vi "Scripting.vi"() -> ()   [LabVIEW 2015]
uses:
  Utils/Cluster.ctl
  <vilib>/Utility/file.llb/Read Delimited Spreadsheet (string).vi
  Users/Sherman/Desktop/BETA_GSCS/Systems/TCS_Link/TCSLINK_global.vi
panel:
  out "Current Lamp cluster":T1
  out "Current Setup Name":string
  out "Setup Names":string[](array[string])
  out "Length of script":dbl
  in  "Script":T2
  out "TCP Response":string
  in  "TCP Connection ID":refnum<k5>
  in  "Current Slit":string
  out "Current Target":cluster{"RA":string, "DEC":string}={"RA"="-00:00:00.00", "DEC"="-00:00:00.00"}
  in  "Custom ROI":cluster{i32, i32, i32, i32, i32, i32}[](array[cluster])
  out "Total Cluster":T3(array[cluster]) {"Configuration"."Select Mode:" items=["Custom", "Imaging", "300 All", "600 UV", "600 Blue", "600 Mid", "600 Red", "1200 m0", "1200 m1", "1200 m2", "1200 m3", "1200 m4", "1200 m5", "1200 m6", "1200 m7", "1200 RESOLVE", "400 m1", "400 m2", "930 m1", "930 m2", "930 m3", "930 m4", "930 m5", "930 m6", "400WD", "930TP", "400Fermi", "400Padgett", "400Lewis", "400Crotts", "600BLee", "600RLee", "400WW"]; "SI camera info"."DomePercent" min=0 step=1; "SI camera info"."Quartz Percent" min=0 step=1; "SI camera info"."CCD Readout Speed" items=["750 kHz, ATTN 0", "750 kHz, ATTN 2", "344 kHz, ATTN 0", "344 kHz, ATTN 3", "100 kHz, ATTN 2", "100 kHz, ATTN 3"]; "SI camera info"."CCD ROI Mode" items=["Imaging, 1x1  "=0, "Imaging, 2x2"=1, "Imaging, 3x3"=2, "Spectroscopic, 1x1"=3, "Spectroscopic, 2x2"=4, "Spectroscopic, 3x3"=5, "MOS, 1x1"=11, "MOS, 2x2"=12, "MOS, 3x3"=13, "Slicer"=6, "Spectroscopic, ZZ Ceti"=14, "Slit Imaging/Alignment"=7, "MOS Imaging/Alignment"=10, "Set user-defined ROI..."=21, "Custom Mode"=9]; "SI camera info"."Number of Exp" min=0 step=1; "SI camera info"."Exp time" min=0 step=1}
  in  "?":T4(tab)
  in  "Shutdown":bool
  in  "Test":bool
  in  "ABORT":bool
  in  "Pause Button":bool
  out "Current Line":dbl caption="Current LIne"
  in  "Make Script":bool
  out "status":string
  in  "Script location":path
  in  "Scripting Active":bool
  out "Runtime":dbl caption="Expected Runtime"
  out "Array":string[](array[string])
  out "Wavelength Mode":string
  out "Secondary Filter":string
  out "Primary Filter":string
  out "Slit":string
  out "Grating":string
  out "Camera Focus":dbl
  out "Grating Angle":dbl
  out "Camera Angle":dbl
  out "Coll Position":dbl
  in  "Get System Info":bool
  in  "Setups":T5(array[cluster])
  # "Eventually Add tcp response to a new tab"
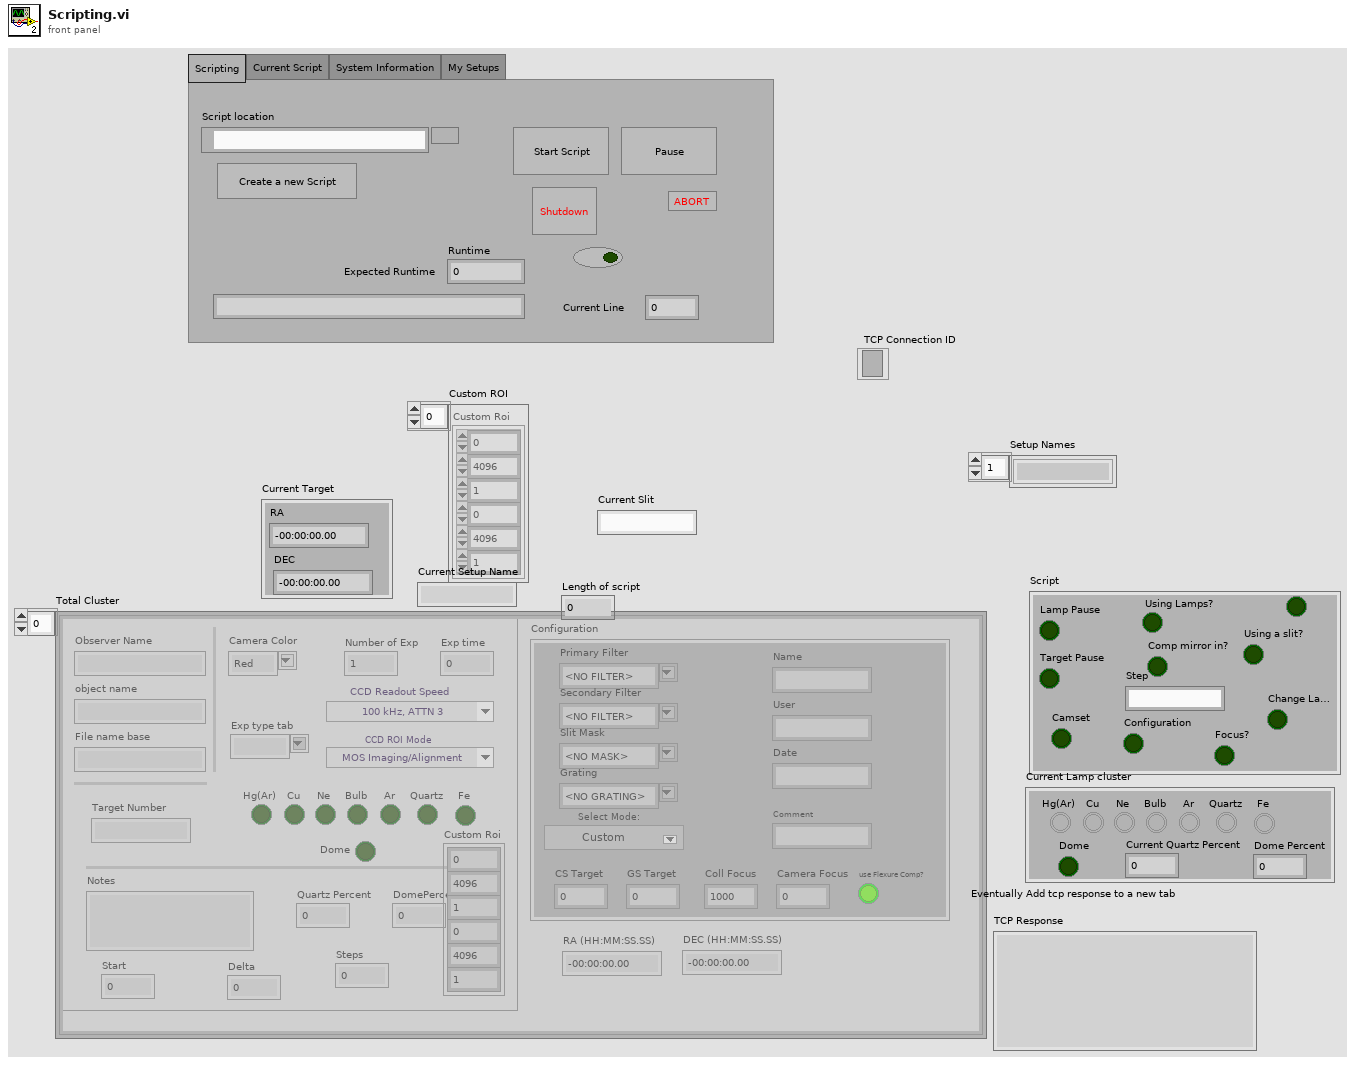
[diagram p1: front panel]
types:
  T1 = cluster{"Bulb":bool, "Fe":bool, "Quartz":bool, "Ar":bool, "Ne":bool, "Cu":bool, "Hg(Ar)":bool, "Current Quartz Percent":dbl, "Dome":bool, "Dome Percent":dbl}
  T2 = cluster{"Lamp Pause":bool, "Target Pause":bool, "Using Lamps?":bool, "Step":string, "Camset":bool, "Configuration":bool, "Using a slit?":bool, "Change Lamps":bool, "Boolean":bool, "Comp mirror in?":bool, "Focus?":bool}
  T3 = cluster{"SI camera info":cluster{"Observer Name":string, "object name":string, "File name base":string, "Camera Color":string, "Exp type tab":string, "Number of Exp":i32, "Exp time":i32, "CCD Readout Speed":u8, "CCD ROI Mode":u16, "Hg(Ar)":bool, "Cu":bool, "Ne":bool, "Bulb":bool, "Ar":bool, "Quartz":bool, "Quartz Percent":i32, "Fe":bool, "Notes":string, "Target Number":string, "DomePercent":i32, "Dome":bool, "Start":dbl, "Delta":dbl, "Steps":dbl, "Custom Roi":cluster{i32, i32, i32, i32, i32, i32}}, "Configuration":cluster{"Primary Filter":string, "Secondary Filter":string, "Slit Mask":string, "Grating":string, "CS Target":dbl, "GS Target":dbl, "Coll Focus":i32, "Camera Focus":i32, "Name":string, "User":string, "Date":string, "Comment":string, "use Flexure Comp?":bool, "Select Mode:":u16}, "RA (HH:MM:SS.SS)":string, "DEC (HH:MM:SS.SS)":string}[]
  T4 = enum32{"Scripting", "Current Script", "System Information", "My Setups"}
  T5 = cluster{"Setup Name":string, "Focus Value":dbl, "Focus Test updated?":bool}[]
  T6 = typedef "Cluster.ctl" = cluster{"SI camera info":cluster{"Observer Name":string, "object name":string, "File name base":string, "Camera Color":string, "Exp type tab":string, "Number of Exp":i32, "Exp time":i32, "CCD Readout Speed":u8, "CCD ROI Mode":u16, "Hg(Ar)":bool, "Cu":bool, "Ne":bool, "Bulb":bool, "Ar":bool, "Quartz":bool, "Quartz Percent":i32, "Fe":bool, "Notes":string, "Target Number":string, "DomePercent":i32, "Dome":bool, "Start":dbl, "Delta":dbl, "Steps":dbl, "Custom Roi":cluster{i32, i32, i32, i32, i32, i32}}, "Configuration":cluster{"Primary Filter":string, "Secondary Filter":string, "Slit Mask":string, "Grating":string, "CS Target":dbl, "GS Target":dbl, "Coll Focus":i32, "Camera Focus":i32, "Name":string, "User":string, "Date":string, "Comment":string, "use Flexure Comp?":bool, "Select Mode:":u16}, "RA (HH:MM:SS.SS)":string, "DEC (HH:MM:SS.SS)":string}
  T7 = cluster{"Setup Name":string, "Camera Focus":dbl, "Focus test updated?":bool}
  T8 = cluster{"SI camera info":cluster{"Observer Name":string, "object name":string, "File name base":string, "Camera Color":string, "Exp type tab":string, "Number of Exp":i32, "Exp time":i32, "CCD Readout Speed":u8, "CCD ROI Mode":u16, "Hg(Ar)":bool, "Cu":bool, "Ne":bool, "Bulb":bool, "Ar":bool, "Quartz":bool, "Quartz Percent":i32, "Fe":bool, "Notes":string, "Target Number":string, "DomePercent":i32, "Dome":bool, "Start":dbl, "Delta":dbl, "Steps":dbl, "Custom Roi":cluster{i32, i32, i32, i32, i32, i32}}, "Configuration":cluster{"Primary Filter":string, "Secondary Filter":string, "Slit Mask":string, "Grating":string, "CS Target":dbl, "GS Target":dbl, "Coll Focus":i32, "Camera Focus":i32, "Name":string, "User":string, "Date":string, "Comment":string, "use Flexure Comp?":bool, "Select Mode:":u16}, "RA (HH:MM:SS.SS)":string, "DEC (HH:MM:SS.SS)":string}
  T9 = cluster{"Setup Name":string, "Focus Value":dbl, "Focus Test updated?":bool}
  T10 = cluster{"Primary Filter":string, "Secondary Filter":string, "Slit Mask":string, "Grating":string, "CS Target":dbl, "GS Target":dbl, "Coll Focus":i32, "Camera Focus":i32, "Name":string, "User":string, "Date":string, "Comment":string, "use Flexure Comp?":bool, "Select Mode:":u16}
  T11 = cluster{"Observer Name":string, "object name":string, "File name base":string, "Camera Color":string, "Exp type tab":string, "Number of Exp":i32, "Exp time":i32, "CCD Readout Speed":u8, "CCD ROI Mode":u16, "Hg(Ar)":bool, "Cu":bool, "Ne":bool, "Bulb":bool, "Ar":bool, "Quartz":bool, "Quartz Percent":i32, "Fe":bool, "Notes":string, "Target Number":string, "DomePercent":i32, "Dome":bool, "Start":dbl, "Delta":dbl, "Steps":dbl, "Custom Roi":cluster{i32, i32, i32, i32, i32, i32}}
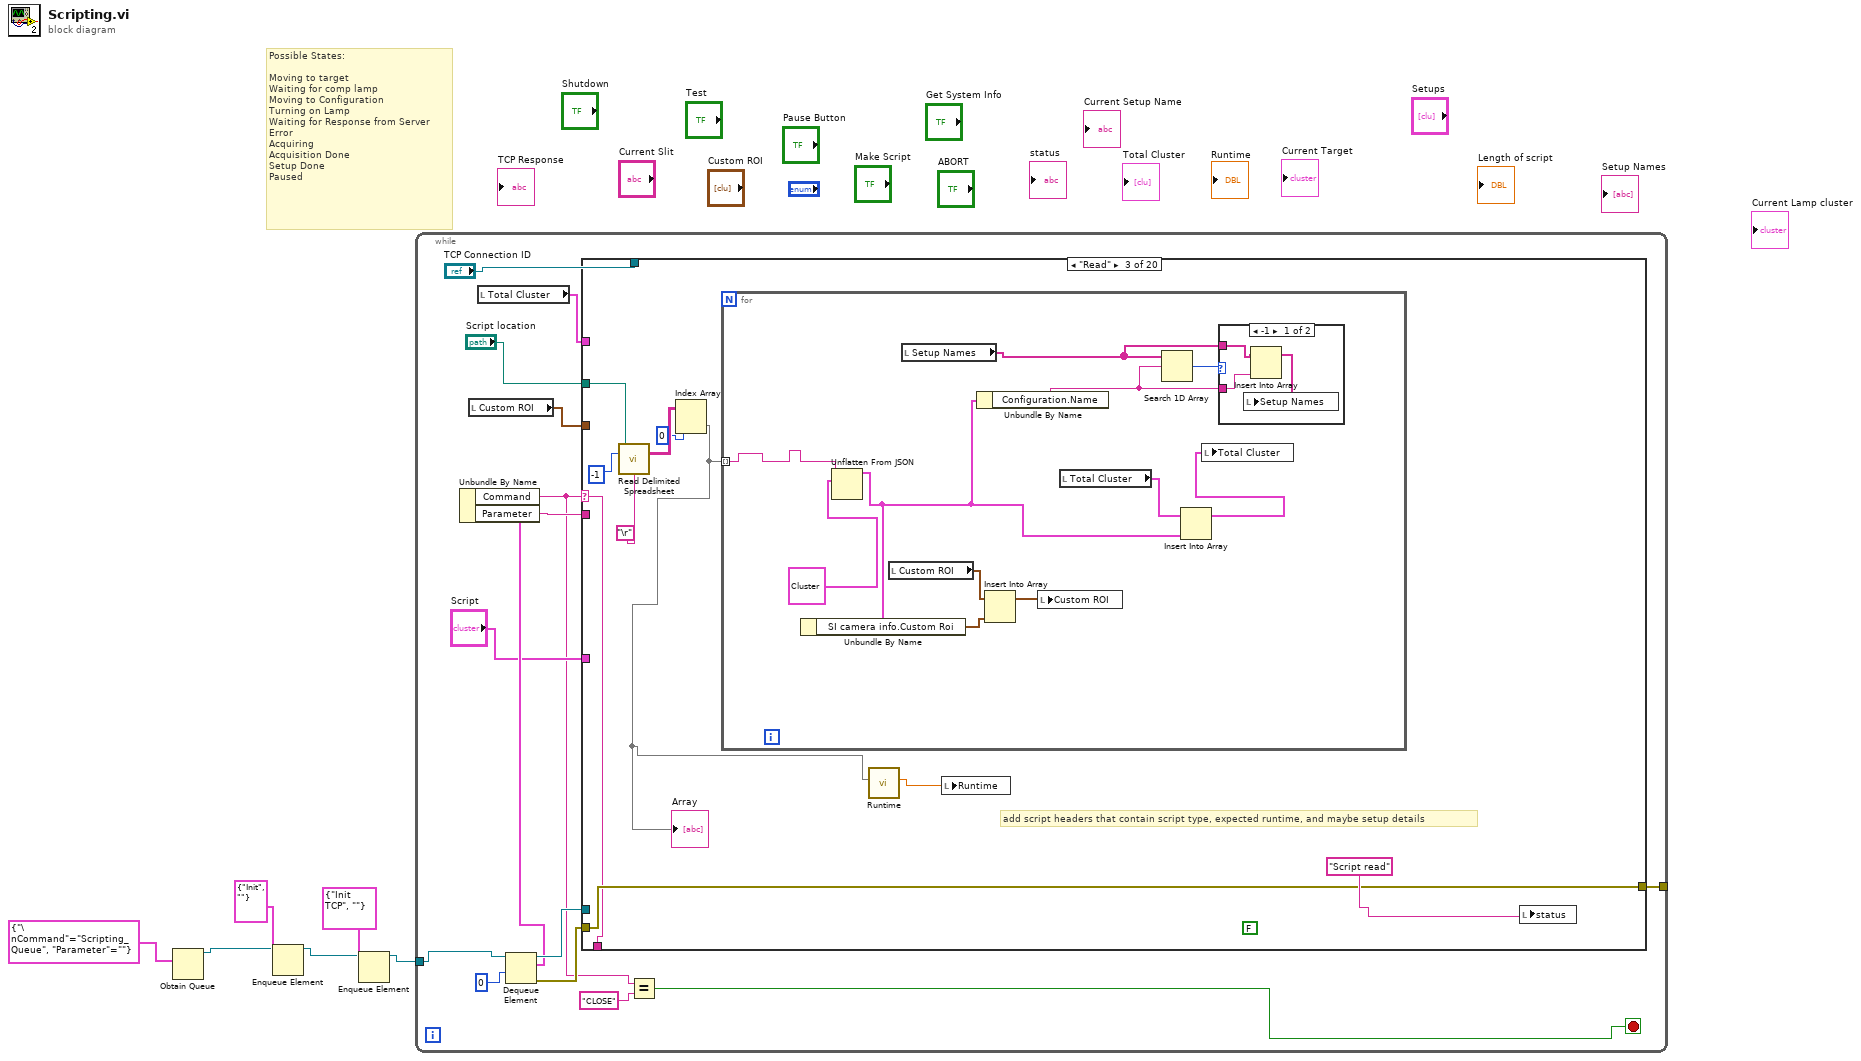
[diagram p0: block diagram]
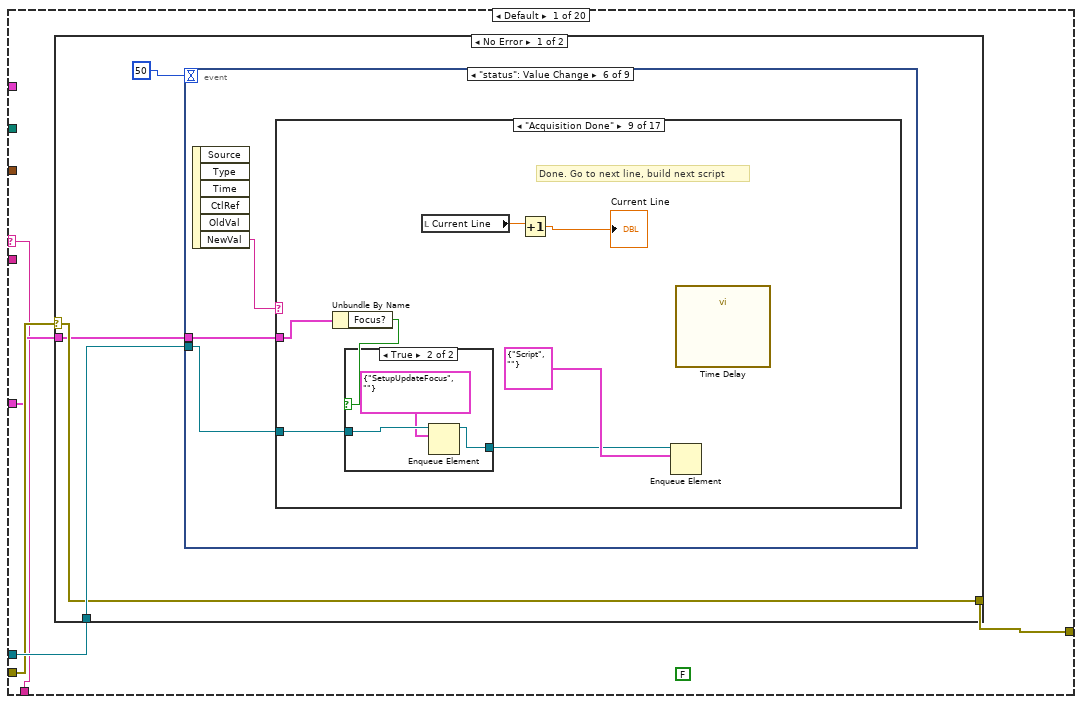
[diagram p2: hidden frame]
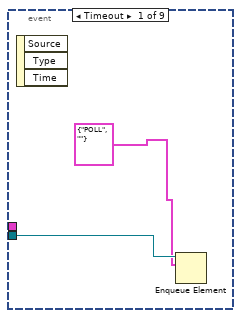
[diagram p3: hidden frame]
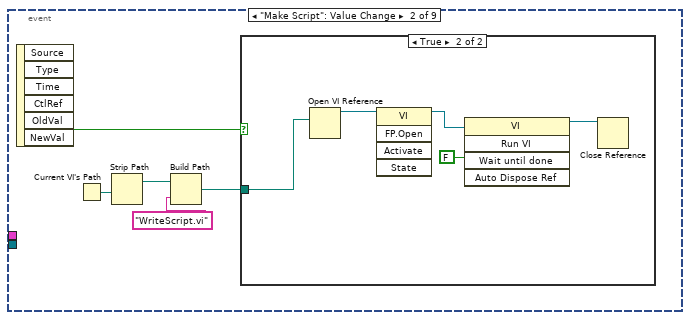
[diagram p4: hidden frame]
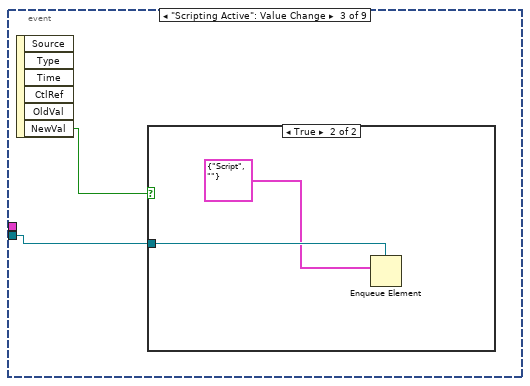
[diagram p6: hidden frame]
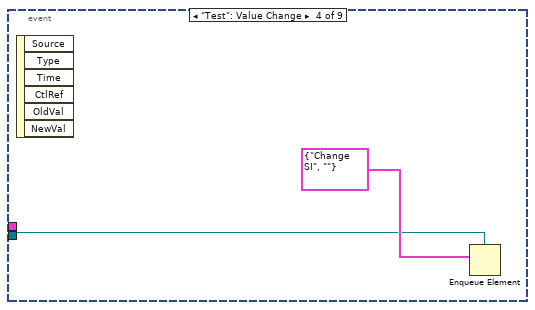
[diagram p8: hidden frame]
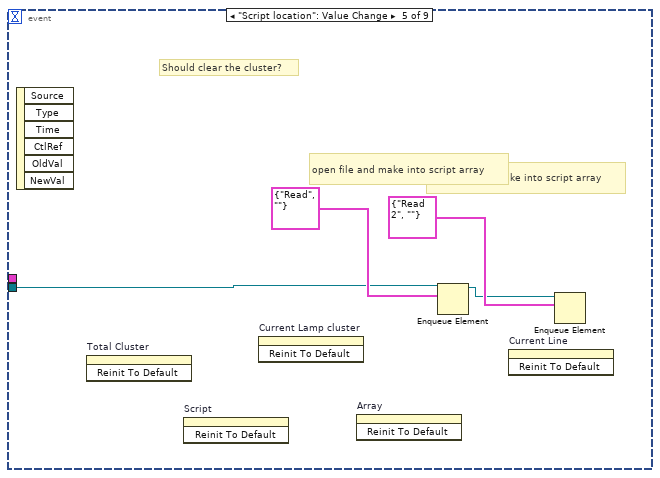
[diagram p9: hidden frame]
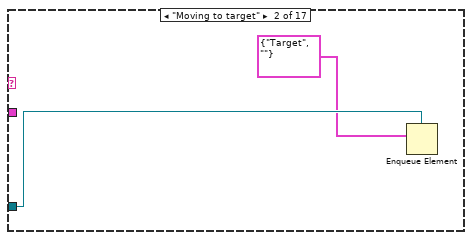
[diagram p11: hidden frame]
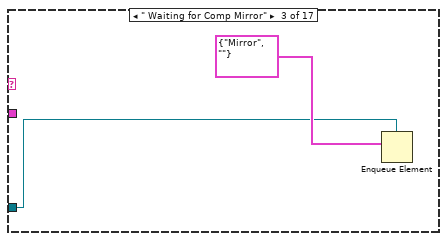
[diagram p12: hidden frame]
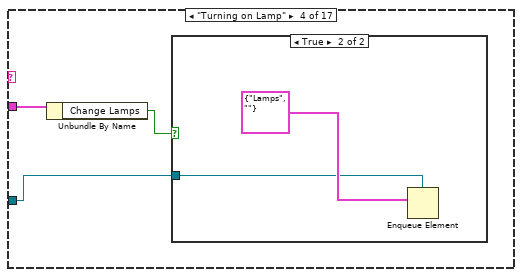
[diagram p13: hidden frame]
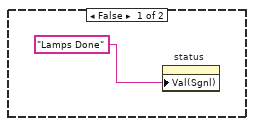
[diagram p14: hidden frame]
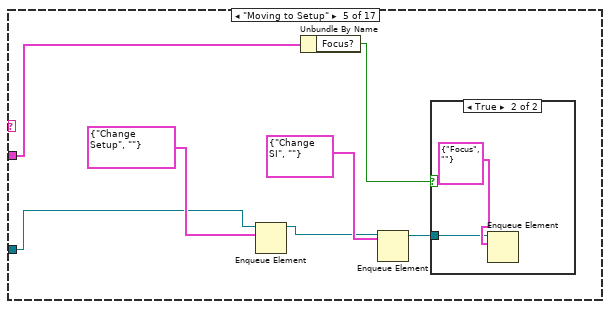
[diagram p15: hidden frame]
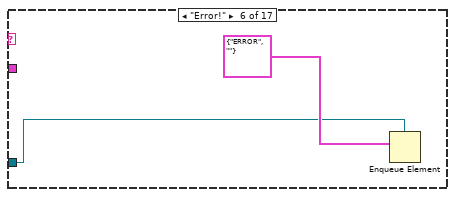
[diagram p17: hidden frame]
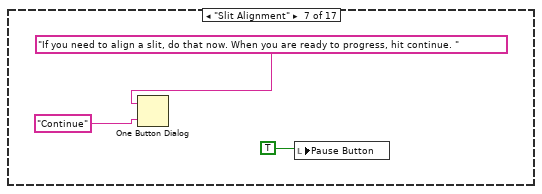
[diagram p18: hidden frame]
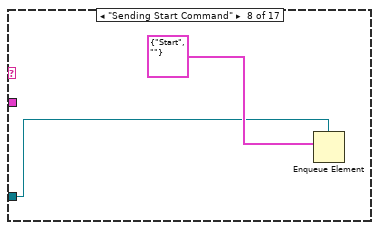
[diagram p19: hidden frame]
diagram:
  # "Possible States:\n\nMoving to target\nWaiting for comp lamp\nMoving to Configuration\nTurning on Lamp\nWaiting for Response from Server\nError\nAcquiring\nAcquisition Done\nSetup Done\nPaused"
  n1 = Obtain Queue(element data type=cluster{"\nCommand":string, "Parameter":string} {"\nCommand"="Scripting_Queue", "Parameter"=""}) -> (queue out=w2:refnum<queue>)  [unwired: 4 in, 2 out]
  n2 = Enqueue Element(queue=w2, element=cluster{string, string} {"Init", ""}) -> (queue out=w1:refnum<queue>)  [unwired: 2 in, 2 out]
  n3 = Enqueue Element(queue=w1, element=cluster{string, string} {"Init TCP", ""}) -> (queue out=w4:refnum<queue>)  [unwired: 2 in, 2 out]
  n4 = while {
    tunnel: w4 -> [w16]
    tunnel: [w11] -> _
    stop <- w7 stop-if-true
    n5 = local read "Custom ROI"() -> (w14:cluster{i32, i32, i32, i32, i32, i32}[])
    n6 = local read "Total Cluster"() -> (w17:T3)
    n7 = Dequeue Element(queue=w16, timeout in ms (-1)=0) -> (queue out=w21:refnum<queue>, element=w20:cluster{"\nCommand":string, "Parameter":string}, error out=w12:errorcluster)  [unwired: 1 in, 1 out]
    n8 = Unbundle By Name(w20) -> ("Command"=w8:string, "Parameter"=w19:string)
    n9 = case shown="\"Read\"" w8 {
      selector: w8 -> [w22 w120 w243 w263 w275 w315 w374 w408 w430 w459 w486 w503 w515 w531 w548 w579 w598 w606 w617 w635]
      tunnel: w21 -> [w26 _ _ _ _ _ _ _ _ _ _ _ _ _ _ _ _ w609 w620 _]
      tunnel: w19 -> [_ _ _ _ _ _ _ _ _ _ _ _ _ _ _ _ _ _ _ _]
      tunnel: "Script location" -> [_ _ w248 _ _ _ _ _ _ _ _ _ _ _ _ _ _ _ _ _]
      tunnel: w17 -> [_ _ _ _ w280 w352 _ w423 w446 w471 w498 _ _ _ _ _ _ _ _ _]
      tunnel: w14 -> [_ _ _ _ _ _ _ _ _ _ _ _ _ _ _ _ _ _ _ _]
      tunnel: "TCP Connection ID" -> [_ w130 _ _ _ w354 w388 w421 w443 w468 w495 _ w518 w534 w551 w587 _ _ _ w636]
      tunnel: w12 -> [w25 w125 w244 w264 w281 w350 w386 w394 w433 w457 w480 w504 w519 w533 w550 w586 w599 w612 w625 w637]
      tunnel: [w24 w127 w244 w264 w281 w353 w387 w420 w431 w460 w487 w504 w516 w535 w552 w588 w599 w610 w619 w638] -> w11
      tunnel: "Script" -> [w23 w128 _ _ _ _ w369 _ _ _ _ _ _ _ _ _ _ _ _ _]
      tunnel: [w22 w120 w243 w263 w275 w315 w374 w408 w430 w459 w486 w503 w515 w531 w548 w579 w598 w606 w617 w635] -> _
      frame Default {
        (unwired) FALSE
        n10 = case shown="No Error" w25 {
          selector: w25 -> [w29 w117]
          tunnel: w26 -> [w30 w118]
          tunnel: [w29 w117] -> w24
          tunnel: w23 -> [w27 _]
          frame No Error {
            n11 = event shown="[5] \"status\": Value Change" {
              selector: _ -> [_ _ _ _ _ _ _ _ _]
              dyn-events: _ -> [_ _ _ _ _ _ _ _ _]
              timeout: 50 -> [_ _ _ _ _ _ _ _ _]
              tunnel: w30 -> [w32 _ w44 w47 w51 w54 w110 w112 w114]
              tunnel: w27 -> [_ _ _ _ _ w53 _ _ _]
              event Timeout {
                n12 = event-data() -> ()  [unwired: 1 in, 3 out]
                n13 = Enqueue Element(queue=w32, element=cluster{string, string} {"POLL", ""}) -> ()  [unwired: 2 in, 3 out]
              }
              event "Make Script": Value Change {
                n14 = event-data() -> ("NewVal"=w37:bool)  [unwired: 1 in, 5 out]
                n15 = Current VI's Path() -> (path=w34:path)
                n16 = Strip Path(path=w34) -> (stripped path=w35:path)  [unwired: 1 out]
                n17 = Build Path(base path=w35, name or relative path="WriteScript.vi") -> (appended path=w33:path)
                n18 = case shown="True" w37 {
                  tunnel: w33 -> [_ w38]
                  frame False {
                  }
                  frame True {
                    n19 = Open VI Reference(vi path=w38) -> (vi reference=w42:refnum<vi>)  [unwired: 5 in, 1 out]
                    n20 = invoke class="VI" method="FP.Open"(reference=w42) -> (reference out=w41:refnum<vi>)  [unwired: 4 in, 4 out]
                    n21 = invoke class="VI" method="Run VI"(reference=w41, "Wait until done"=FALSE) -> (reference out=w39:refnum<vi>)  [unwired: 3 in, 4 out]
                    n22 = Close Reference(reference=w39) -> ()  [unwired: 1 in, 1 out]
                  }
                }
              }
              event "Scripting Active": Value Change {
                n23 = event-data() -> ("NewVal"=w43:bool)  [unwired: 1 in, 5 out]
                n24 = case shown="True" w43 {
                  tunnel: w44 -> [_ w46]
                  frame False {
                  }
                  frame True {
                    n25 = Enqueue Element(queue=w46, element=cluster{string, string} {"Script", ""}) -> ()  [unwired: 2 in, 3 out]
                  }
                }
              }
              event "Test": Value Change {
                n26 = event-data() -> ()  [unwired: 1 in, 6 out]
                n27 = Enqueue Element(queue=w47, element=cluster{string, string} {"Change SI", ""}) -> ()  [unwired: 2 in, 3 out]
              }
              event "Script location": Value Change {
                # "open file and make into script array"
                # "Should clear the cluster?"
                # "open file and make into script array"
                n28 = event-data() -> ()  [unwired: 1 in, 6 out]
                n29 = invoke on="Total Cluster" class="Arr (strict)" method="Reinit To Default"() -> ()  [unwired: 3 in, 3 out]
                n30 = invoke on="Script" class="Clust (strict)" method="Reinit To Default"() -> ()  [unwired: 3 in, 3 out]
                n31 = invoke on="Current Lamp cluster" class="Clust (strict)" method="Reinit To Default"() -> ()  [unwired: 3 in, 3 out]
                n32 = invoke on="Array" class="Arr (strict)" method="Reinit To Default"() -> ()  [unwired: 3 in, 3 out]
                n33 = Enqueue Element(queue=w51, element=cluster{string, string} {"Read", ""}) -> (queue out=w49:refnum<queue>)  [unwired: 2 in, 2 out]
                n34 = invoke on="Current Line" class="DigNum (strict)" method="Reinit To Default"() -> ()  [unwired: 3 in, 3 out]
                n35 = Enqueue Element(queue=w49, element=cluster{string, string} {"Read 2", ""}) -> ()  [unwired: 2 in, 3 out]
              }
              event "status": Value Change {
                n36 = event-data() -> ("NewVal"=w55:string)  [unwired: 1 in, 5 out]
                n37 = case shown="\"Acquisition Done\"" w55 {
                  tunnel: w54 -> [_ w57 w58 w62 w71 w75 _ w80 w83 _ _ _ _ _ _ _ w108]
                  tunnel: w53 -> [_ _ _ w61 w67 _ _ _ w85 _ _ _ _ _ _ _ _]
                  frame "", Default {
                    # "Possible States:\n\nMoving to target\nWaiting for comp lamp\nMoving to Configuration\nTurning on Lamp\nWaiting for Response from Server\nError\nExposing\nExposure Done\nSetup Done\nPaused"
                  }
                  frame "Moving to target" {
                    n38 = Enqueue Element(queue=w57, element=cluster{string, string} {"Target", ""}) -> ()  [unwired: 2 in, 3 out]
                  }
                  frame " Waiting for Comp Mirror" {
                    n39 = Enqueue Element(queue=w58, element=cluster{string, string} {"Mirror", ""}) -> ()  [unwired: 2 in, 3 out]
                  }
                  frame "Turning on Lamp" {
                    n40 = Unbundle By Name(w61) -> ("Change Lamps"=w60:bool)
                    n41 = case shown="True" w60 {
                      tunnel: w62 -> [_ w64]
                      frame False {
                        n42 = property on="status" class="Str"("Val(Sgnl)"="Lamps Done") -> ()  [unwired: 2 in, 2 out]
                      }
                      frame True {
                        n43 = Enqueue Element(queue=w64, element=cluster{string, string} {"Lamps", ""}) -> ()  [unwired: 2 in, 3 out]
                      }
                    }
                  }
                  frame "Moving to Setup" {
                    n44 = Enqueue Element(queue=w71, element=cluster{string, string} {"Change Setup", ""}) -> (queue out=w69:refnum<queue>)  [unwired: 2 in, 2 out]
                    n45 = Unbundle By Name(w67) -> ("Focus?"=w66:bool)
                    n46 = Enqueue Element(queue=w69, element=cluster{string, string} {"Change SI", ""}) -> (queue out=w68:refnum<queue>)  [unwired: 2 in, 2 out]
                    n47 = case shown="True" w66 {
                      tunnel: w68 -> [_ w73]
                      frame False {
                      }
                      frame True {
                        n48 = Enqueue Element(queue=w73, element=cluster{string, string} {"Focus", ""}) -> ()  [unwired: 2 in, 3 out]
                      }
                    }
                  }
                  frame "Error!" {
                    n49 = Enqueue Element(queue=w75, element=cluster{string, string} {"ERROR", ""}) -> ()  [unwired: 2 in, 3 out]
                  }
                  frame "Slit Alignment" {
                    n50 = One Button Dialog(message="If you need to align a slit, do that now. When you are ready to progress, hit continue. ", button name ("OK")="Continue") -> ()  [unwired: 1 out]
                    n51 = local write "Pause Button"(TRUE) -> ()
                  }
                  frame "Sending Start Command" {
                    n52 = Enqueue Element(queue=w80, element=cluster{string, string} {"Start", ""}) -> ()  [unwired: 2 in, 3 out]
                  }
                  frame "Acquisition Done" {
                    # "Done. Go to next line, build next script"
                    n53 = Unbundle By Name(w85) -> ("Focus?"=w84:bool)
                    n54 = case shown="True" w84 {
                      tunnel: w83 -> [w89 w91]
                      tunnel: [w89 w92] -> w82
                      frame False {
                      }
                      frame True {
                        n55 = Enqueue Element(queue=w91, element=cluster{string, string} {"SetupUpdateFocus", ""}) -> (queue out=w92:refnum<queue>)  [unwired: 2 in, 2 out]
                      }
                    }
                    n56 = local read "Current Line"() -> (w88:dbl)
                    n57 = Increment(x=w88) -> (x+1=→"Current Line":dbl)
                    n58 = Enqueue Element(queue=w82, element=cluster{string, string} {"Script", ""}) -> ()  [unwired: 2 in, 3 out]
                    n59 = call "Time Delay"() -> ()  [unwired: 11 in, 1 out]
                  }
                  frame "Abort Done" {
                    n60 = local write "Scripting Active"(FALSE) -> ()
                  }
                  frame "Setup Done" {
                    n61 = local read "Script"() -> (w95:T2)
                    n62 = Bundle By Name(cluster=w95, "Configuration"=TRUE) -> (w94:T2)
                    n63 = local write "Script"(w94) -> ()
                  }
                  frame "Camera setup Done" {
                    n64 = local read "Script"() -> (w99:T2)
                    n65 = Bundle By Name(cluster=w99, "Camset"=TRUE) -> (w98:T2)
                    n66 = local write "Script"(w98) -> ()
                  }
                  frame "Moved to Target" {
                    n67 = local read "Script"() -> (w102:T2)
                    n68 = Bundle By Name(cluster=w102, "Step"="Moved to Target") -> (w101:T2)
                    n69 = local write "Script"(w101) -> ()
                  }
                  frame "Paused" {
                  }
                  frame "Lamps Done" {
                    # "Fe is the last lamp. Once this one is done then all lamps should be done"
                    n70 = local read "Script"() -> (w105:T2)
                    n71 = Bundle By Name(cluster=w105, "Step"="Acquire") -> (w104:T2)
                    n72 = local write "Script"(w104) -> ()
                  }
                  frame "Script Complete" {
                    n73 = property on="Scripting Active" class="Bool (strict)"("Value"=FALSE) -> ()  [unwired: 2 in, 2 out]
                  }
                  frame "Shutdown Complete" {
                    n74 = Enqueue Element(queue=w108, element=cluster{string, string} {"CLOSE", ""}) -> ()  [unwired: 2 in, 3 out]
                  }
                }
              }
              event "ABORT": Value Change {
                n75 = event-data() -> ()  [unwired: 1 in, 6 out]
                n76 = local write "status"("Aborting") -> ()
                n77 = Enqueue Element(queue=w110, element=cluster{string, string} {"Abort", ""}) -> ()  [unwired: 2 in, 3 out]
              }
              event "Shutdown": Value Change {
                n78 = event-data() -> ()  [unwired: 1 in, 6 out]
                n79 = Enqueue Element(queue=w112, element=cluster{string, string} {"SHUTDOWN", ""}) -> ()  [unwired: 2 in, 3 out]
              }
              event "Get System Info": Value Change {
                n80 = event-data() -> ()  [unwired: 1 in, 6 out]
                n81 = Enqueue Element(queue=w114, element=cluster{string, string} {"SYSTEM_POS", ""}) -> ()  [unwired: 2 in, 3 out]
              }
            }
          }
          frame Error {
            # "Stop"
            n82 = local write "Pause Button"(TRUE) -> ()
            n83 = Enqueue Element(queue=w118, element=cluster{string, string} {"ERROR", ""}) -> ()  [unwired: 2 in, 3 out]
          }
        }
      }
      frame "POLL" {
        (unwired) FALSE
        # "precheck\nmove to setup\ntarget\nslit\nlamps\ngo"
        # "govern pauses"
        # "Or skip line or repeat line"
        # "When IMAGINGDONE is recieved +1"
        # "Paused?"
        # "TCP/IP Reads"
        # "3. wait for all commands are recieved as done"
        # "2.5  turn on lamp"
        # "4. Once Setup, SI params, and user input: start exposure"
        # "2. Move to Setup\nand Si params"
        # "2. If changing targets, or if going from no \nlamps to lamp, wait for user input"
        # "1. Check current lamp/current target"
        # "get responses on commands and update status"
        n84 = call "TCP Read with Size.vi"("error in (no error)"=w125, "timeout ms (25000)"=1000, "connection ID"=w130) -> ("error out"=w126:errorcluster, "data out"=w123:string)  [unwired: 6 in, 1 out]
        n85 = case shown="Error" w126 {
          selector: w126 -> [w132 w133]
          tunnel: [w132 w134] -> w124
          frame No Error {
          }
          frame Error {
            n86 = Unbundle By Name(w133) -> ("code"=w135:i32)
            n87 = case shown="56" w135 {
              tunnel: [w136 errorcluster {"status"=FALSE, "code"=0, "source"=""} ("error constant")] -> w134
              tunnel: w133 -> [w136 _]
              frame 0, Default {
              }
              frame 56 {
              }
            }
          }
        }
        n88 = call "ParseCommand2.vi"("Command string"=w123) -> ("Command"=w122:string, "Parameters"=w121:string[])
        n89 = case shown="False" "Scripting Active" {
          tunnel: w128 -> [_ w138]
          frame False {
            # "Script is not Active"
          }
          frame True {
            n90 = local read "Pause Button"() -> (w139:bool)
            n91 = case shown="False" w139 {
              tunnel: w138 -> [w147 _]
              frame False {
                # "Scripting is on and we arent paused. Attempt to progress through Script"
                n92 = Unbundle By Name(w147) -> ("Step"=w146:string, "Target Pause"=w145:bool, "Using Lamps?"=w144:bool, "Lamp Pause"=w143:bool, "Camset"=w142:bool, "Configuration"=w141:bool, "Using a slit?"=w140:bool)
                n93 = case shown="\"Ordered Moves\"" w146 {
                  tunnel: w145 -> [_ _ _ w158 _ _ _ _]
                  tunnel: w144 -> [_ _ _ _ w163 w176 _ _]
                  tunnel: w143 -> [_ _ _ _ _ w177 _ _]
                  tunnel: w142 -> [_ _ w154 _ _ _ _ _]
                  tunnel: w141 -> [_ _ w153 _ _ _ _ _]
                  tunnel: w140 -> [_ _ _ _ w164 _ _ _]
                  frame "", Default {
                  }
                  frame "Precheck Run" {
                    n94 = property on="status" class="Str"("Val(Sgnl)"="Moving to Setup") -> ()  [unwired: 2 in, 2 out]
                    n95 = local read "Script"() -> (w149:T2)
                    n96 = Bundle By Name(cluster=w149, "Step"="Ordered Moves") -> (w148:T2)
                    n97 = local write "Script"(w148) -> ()
                  }
                  frame "Ordered Moves" {
                    # "wait to get dones from both"
                    n98 = And(x=w154, y=w153) -> (x .and. y?=w152:bool)
                    n99 = case shown="False" w152 {
                      frame False {
                        # "keep waiting"
                      }
                      frame True {
                        n100 = local read "Script"() -> (w155:T2)
                        n101 = Bundle By Name(cluster=w155, "Step"="Moved to Setup") -> (w156:T2)
                        n102 = local write "Script"(w156) -> ()
                      }
                    }
                  }
                  frame "Moved to Setup" {
                    n103 = case shown="True" w158 {
                      frame False {
                        n104 = local read "Script"() -> (w160:T2)
                        n105 = Bundle By Name(cluster=w160, "Step"="Moved to Target") -> (w159:T2)
                        n106 = local write "Script"(w159) -> ()
                      }
                      frame True {
                        n107 = property on="status" class="Str"("Val(Sgnl)"="Moving to target") -> ()  [unwired: 2 in, 2 out]
                      }
                    }
                  }
                  frame "Moved to Target" {
                    n108 = case shown="False" w164 {
                      tunnel: w163 -> [_ w168]
                      frame False {
                        n109 = local read "Script"() -> (w167:T2)
                        n110 = Bundle By Name(cluster=w167, "Step"="Lamps") -> (w166:T2)
                        n111 = local write "Script"(w166) -> ()
                      }
                      frame True {
                        n112 = case shown="True" w168 {
                          frame False {
                            # "slit no lamp= need to align slit"
                            n113 = property on="status" class="Str"("Val(Sgnl)"="Slit Alignment") -> ()  [unwired: 2 in, 2 out]
                            n114 = local read "Script"() -> (w169:T2)
                            n115 = Bundle By Name(cluster=w169, "Step"="Lamps") -> (w170:T2)
                            n116 = local write "Script"(w170) -> ()
                          }
                          frame True {
                            # "If using slit and lamp, just doing callibrations"
                            n117 = local read "Script"() -> (w173:T2)
                            n118 = Bundle By Name(cluster=w173, "Step"="Lamps") -> (w174:T2)
                            n119 = local write "Script"(w174) -> ()
                          }
                        }
                      }
                    }
                  }
                  frame "Lamps" {
                    n120 = case shown="True" w177 {
                      tunnel: w176 -> [w178 _]
                      frame False {
                        n121 = case shown="True" w178 {
                          frame False {
                            n122 = local read "Script"() -> (w179:T2)
                            n123 = Bundle By Name(cluster=w179, "Step"="Acquire") -> (w180:T2)
                            n124 = local write "Script"(w180) -> ()
                          }
                          frame True {
                            n125 = property on="status" class="Str"("Val(Sgnl)"="Turning on Lamp") -> ()  [unwired: 2 in, 2 out]
                            n126 = local read "Script"() -> (w183:T2)
                            n127 = Bundle By Name(cluster=w183, "Step"="Acquire") -> (w184:T2)
                            n128 = local write "Script"(w184) -> ()
                          }
                        }
                      }
                      frame True {
                        n129 = property on="status" class="Str"("Val(Sgnl)"=" Waiting for Comp Mirror") -> ()  [unwired: 2 in, 2 out]
                      }
                    }
                  }
                  frame "Acquire" {
                    n130 = property on="status" class="Str"("Val(Sgnl)"="Sending Start Command") -> ()  [unwired: 2 in, 2 out]
                    n131 = local read "Script"() -> (w188:T2)
                    n132 = Bundle By Name(cluster=w188, "Step"="Exposure Active") -> (w189:T2)
                    n133 = local write "Script"(w189) -> ()
                  }
                  frame "Exposure Active" {
                    # "Just sitting waiting for IMAGINGDONE"
                  }
                }
              }
              frame True {
                # "Either Paused or there was an error that forced a pause"
              }
            }
          }
        }
        n134 = case shown="\"\", Default" w122 {
          tunnel: w121 -> [_ w195 w221 w233]
          tunnel: [w191 w192 w220 w229] -> w127
          tunnel: w124 -> [w191 w192 w220 _]
          frame "", Default {
            # "probably time out"
          }
          frame "DONE" {
            # "Param X was Done"
            n135 = Index Array(array=w195) -> (element=w194:string)  [unwired: 1 in]
            n136 = case shown="\"CAMSET\"" w194 {
              selector: w194 -> [w201 _ _ _ _ _ _]
              tunnel: [w200 "Setup Done" "Moved to Target" "Shutdown Complete" "Setup Done" "Camera setup Done" "Abort Done"] -> w193
              frame "", Default {
                n137 = call <vilib>:"Space Constant.vi"() -> ("String"=w198:string)
                n138 = Concatenate Strings(w201, w198, "Done") -> (w200:string)
              }
              frame "SETUP" {
                n139 = local read "Script"() -> (w203:T2)
                n140 = Bundle By Name(cluster=w203, "Configuration"=TRUE) -> (w202:T2)
                n141 = local write "Script"(w202) -> ()
              }
              frame "TARGET" {
              }
              frame "Shutdown" {
              }
              frame "SETUPNOCHANGE" {
                n142 = local read "Script"() -> (w209:T2)
                n143 = Bundle By Name(cluster=w209, "Configuration"=TRUE) -> (w210:T2)
                n144 = local write "Script"(w210) -> ()
              }
              frame "CAMSET" {
                n145 = local read "Script"() -> (w212:T2)
                n146 = Bundle By Name(cluster=w212, "Camset"=TRUE) -> (w214:T2)
                n147 = local write "Script"(w214) -> ()
              }
              frame "ABORT" {
              }
            }
            n148 = for {
              tunnel: w195 -> [w218] mode=indexing
              shift-right: [w217] -> w196
              shift-left: "" -> [w219]
              n149 = Concatenate Strings(w219, w218) -> (w217:string)
            }
            n150 = property on="status" class="Str"("Val(Sgnl)"=w193) -> ()  [unwired: 2 in, 2 out]
            n151 = local write "TCP Response"(w196) -> ()
          }
          frame "STATUS" {
            n152 = Array Size(array=w221) -> (size(s)=w222:i32)
            n153 = case shown="1" w222 {
              tunnel: w221 -> [_ w224]
              frame 0, Default {
                # "must be syspos or sys status"
              }
              frame 1 {
                n154 = Index Array(array=w224) -> (element=w223:string)  [unwired: 1 in]
                n155 = case shown="\"IMAGINGDONE\"" w223 {
                  frame "IMAGINGDONE" {
                    n156 = property on="status" class="Str"("Val(Sgnl)"="Acquisition Done") -> ()  [unwired: 2 in, 2 out]
                  }
                  frame "", Default {
                  }
                  frame "IMAGING" {
                    n157 = property on="status" class="Str"("Val(Sgnl)"="Acquiring") -> ()  [unwired: 2 in, 2 out]
                  }
                }
              }
            }
          }
          frame "ERROR" {
            # "pause = T"
            n158 = for {
              tunnel: w233 -> [w237] mode=indexing
              shift-right: [w236] -> w228
              shift-left: "" -> [w238]
              n159 = Concatenate Strings(w238, w237) -> (w236:string)
            }
            n160 = property on="status" class="Str"("Val(Sgnl)"="Error!") -> ()  [unwired: 2 in, 2 out]
            n161 = local write "TCP Response"(w228) -> ()
            n162 = local write "Pause Button"(TRUE) -> ()
            n163 = Bundle By Name(cluster=errorcluster {"status"=TRUE, "code"=0, "source"=""} ("error constant"), "status"=TRUE, "code"=0, "source"=w228) -> (w229:errorcluster)
          }
        }
      }
      frame "Read" {
        (unwired) FALSE
        # "add script headers that contain script type, expected runtime, and maybe setup details"
        n164 = call-poly <vilib>:"Read Delimited Spreadsheet.vi"("file path (dialog if empty)"=w248, "number of rows (all:-1)"=-1, "delimiter (\\t)"="\r") -> ("all rows"=w242:string[][])  [unwired: 7 in, 5 out]
        n165 = Index Array(array=w242, index (col)=0) -> (element=w240:string[])  [unwired: 1 in]
        "Array" <- w240
        n166 = for {
          tunnel: w240 -> [w259] mode=indexing
          n167 = Unflatten From JSON(JSON string=w259, type and defaults=T6 {"SI camera info"={"Observer Name"="", "object name"="", "File name base"="", "Camera Color"="Blue", "Exp type tab"="Focus", "Number of Exp"=1, "Exp time"=0, "CCD Readout Speed"=5, "CCD ROI Mode"=10, "Hg(Ar)"=FALSE, "Cu"=FALSE, "Ne"=FALSE, "Bulb"=FALSE, "Ar"=FALSE, "Quartz"=FALSE, "Quartz Percent"=0, "Fe"=FALSE, "Notes"="", "Target Number"="", "DomePercent"=0, "Dome"=FALSE, "Start"=0.0, "Delta"=0.0, "Steps"=0.0, "Custom Roi"={0, 4096, 1, 0, 4096, 1}}, "Configuration"={"Primary Filter"="<NO FILTER>", "Secondary Filter"="<NO FILTER>", "Slit Mask"="<NO MASK>", "Grating"="<NO GRATING>", "CS Target"=0.0, "GS Target"=0.0, "Coll Focus"=1000, "Camera Focus"=0, "Name"="tree", "User"="", "Date"="", "Comment"="", "use Flexure Comp?"=TRUE, "Select Mode:"=0}, "RA (HH:MM:SS.SS)"="-00:00:00.00", "DEC (HH:MM:SS.SS)"="-00:00:00.00"} ("cluster")) -> (value=w250:T6)  [unwired: 5 in, 1 out]
          n168 = Unbundle By Name(w250) -> ("SI camera info.Custom Roi"=w249:cluster{i32, i32, i32, i32, i32, i32})
          n169 = local read "Custom ROI"() -> (w258:cluster{i32, i32, i32, i32, i32, i32}[])
          n170 = local read "Setup Names"() -> (w252:string[])
          n171 = Unbundle By Name(w250) -> ("Configuration.Name"=w253:string)
          n172 = Insert Into Array(array=w258, new element=w249) -> (w257:cluster{i32, i32, i32, i32, i32, i32}[])  [unwired: 1 in]
          n173 = local write "Custom ROI"(w257) -> ()
          n174 = local read "Total Cluster"() -> (w255:T3)
          n175 = Search 1D Array(1D array=w252, element=w253) -> (index of element=w254:i32)  [unwired: 1 in]
          n176 = Insert Into Array(array=w255, new element=w250) -> (w256:T3)  [unwired: 1 in]
          n177 = local write "Total Cluster"(w256) -> ()
          n178 = case shown="-1" w254 {
            tunnel: w253 -> [w261 _]
            tunnel: w252 -> [w260 _]
            frame -1 {
              n179 = Insert Into Array(array=w260, new element=w261) -> (w262:string[])  [unwired: 1 in]
              n180 = local write "Setup Names"(w262) -> ()
            }
            frame 0, Default {
              # "Only add new\nsetup names"
            }
          }
        }
        n181 = call "Runtime.vi"("Script"=w240) -> ("Runtime"=w239:dbl)  [unwired: 10 in]
        n182 = local write "Runtime"(w239) -> ()
        n183 = local write "status"("Script read") -> ()
      }
      frame "Read 2" {
        (unwired) FALSE
        n184 = local read "Setup Names"() -> (w267:string[])
        n185 = local read "Total Cluster"() -> (w269:T3)
        n186 = Array Size(array=w269) -> (size(s)=w268:i32)
        n187 = local write "Length of script"(w268) -> ()
        n188 = local read "Setups"() -> (w266:T5)
        n189 = for {
          tunnel: w267 -> [w274] mode=indexing
          shift-right: [w270] -> w265
          shift-left: w266 -> [w272]
          n190 = Bundle By Name(cluster=T7 {"Setup Name"="", "Camera Focus"=0.0, "Focus test updated?"=FALSE}, "Setup Name"=w274) -> (w271:T7)
          n191 = Insert Into Array(array=w272, new element=w271) -> (w270:T5)  [unwired: 1 in]
        }
        n192 = local write "Setups"(w265) -> ()
      }
      frame "Script" {
        (unwired) FALSE
        # "if next line is empty, script is done"
        n193 = local read "Current Line"() -> (w279:dbl)
        n194 = local read "Length of script"() -> (w278:dbl)
        n195 = Greater Or Equal?(x=w279, y=w278) -> (x >= y?=w277:bool)
        n196 = case shown="False" w277 {
          tunnel: [_ w302] -> w276
          tunnel: w280 -> [_ w299]
          tunnel: w279 -> [_ w290]
          frame True {
            # "script is done"
            n197 = property on="status" class="Str"("Val(Sgnl)"="Script Complete") -> ()  [unwired: 2 in, 2 out]
          }
          frame False {
            w300 = FALSE
            # "check if setup has  changed\nor is the first line"
            n198 = local read "Current Setup Name"() -> (w295:string)
            n199 = Index Array(array=w299, index=w290) -> (element=w287:T8)
            n200 = Unbundle By Name(w287) -> ("SI camera info.Exp type tab"=w286:string)
            n201 = Unbundle By Name(w287) -> ("Configuration.Name"=w293:string)
            n202 = local read "Current Lamp cluster"() -> (w291:T1)
            n203 = local read "Current Target"() -> (w283:cluster{"RA":string, "DEC":string})
            n204 = property on="Using Lamps?" class="Bool (strict)"() -> ("Value"=w306:bool)  [unwired: 2 in, 2 out]
            n205 = Equal?(x=w290, y=0) -> (x = y?=w294:bool)
            n206 = case shown="True" w294 {
              tunnel: w293 -> [_ w307]
              frame False {
              }
              frame True {
                n207 = local write "Current Setup Name"(w307) -> ()
              }
            }
            n208 = Equal?(x=w293, y=w295) -> (x = y?=w297:bool)
            n209 = call "Precheck.vi"("Using Lamps"=w306, "Current Lamp cluster"=w291, "Target info"=w283, "cluster"=w287, "line number"=w290) -> ("Comp Mirror in?"=w288:bool, "Lamp Pause"=w303:bool, "Target Pause"=w289:bool, "Change Lamps"=w292:bool, "Using Lamps Out"=w304:bool)  [unwired: 2 in]
            n210 = Or(x=w297, y=w294) -> (x .or. y?=w296:bool)
            n211 = Equal?(x=w286, y="Focus") -> (x = y?=w284:bool)
            n212 = case shown="False" w296 {
              tunnel: w293 -> [w308 _]
              frame False {
                # "make new setup current"
                n213 = local write "Current Setup Name"(w308) -> ()
              }
              frame True {
                # "still on the same setup, \nnothing to do here"
              }
            }
            n214 = local read "Script"() -> (w305:T2)
            n215 = Bundle By Name(cluster=w305, "Target Pause"=w289, "Lamp Pause"=w303, "Using Lamps?"=w304, "Step"="Precheck Run", "Camset"=w300, "Configuration"=w300, "Using a slit?"=w300, "Change Lamps"=w292, "Comp mirror in?"=w288, "Focus?"=w284) -> (w302:T2)
          }
        }
        n216 = local write "Script"(w276) -> ()
      }
      frame "Lamps" {
        (unwired) FALSE
        # "Wait for acknowledgement"
        # "Send to server"
        n217 = local read "Current Line"() -> (w351:dbl)
        n218 = Index Array(array=w352, index=w351) -> (element=w325:T8)
        n219 = Unbundle By Name(w325) -> ("SI camera info.Hg(Ar)"=w340:bool, "SI camera info.Cu"=w339:bool, "SI camera info.Ne"=w338:bool, "SI camera info.Bulb"=w337:bool, "SI camera info.Ar"=w336:bool, "SI camera info.Fe"=w335:bool, "SI camera info.Quartz"=w334:bool, "SI camera info.Dome"=w311:bool, "SI camera info.Quartz Percent"=w314:i32, "SI camera info.DomePercent"=w313:i32)
        n220 = Number To Fractional String(number=w313) -> (F-format string=w312:string)  [unwired: 3 in]
        n221 = Number To Fractional String(number=w314) -> (F-format string=w331:string)  [unwired: 3 in]
        n222 = Build Array(w340, w339, w338, w337, w336, w335, w334, w311) -> (w333:bool[])
        n223 = for {
          tunnel: w333 -> [w361] mode=indexing
          shift-right: [w356] -> w330
          shift-left: string[] [""] -> [w357]
          i -> [w355]
          n224 = Select(t="ON", s=w361, f="OFF") -> (s? t:f=w358:string)
          n225 = Insert Into Array(array=w357, index=w355, new element=w358) -> (w356:string[])
        }
        n226 = Insert Into Array(array=w330, new element #1=w331, new element #2=w312) -> (w328:string[])  [unwired: 1 in]
        n227 = call "FormCommand2.vi"("Parameters"=w328, "Command"="LAMPS") -> ("Command string"=w327:string)
        n228 = call "TCP Write with Size.vi"("error in (no error)"=w350, "data in"=w327, "connection ID"=w354) -> ("error out"=w346:errorcluster, "connection ID out"=w347:refnum<k5>)  [unwired: 6 in, 1 out]
        n229 = call "TCP Read with Size.vi"("error in (no error)"=w346, "timeout ms (25000)"=2000, "connection ID"=w347) -> ("error out"=w341:errorcluster, "data out"=w348:string)  [unwired: 6 in, 1 out]
        n230 = call "ParseCommand.vi"("Command string"=w348) -> ("Command"=w343:string, "Parameters"=w345:string[])
        n231 = Equal?(x="OK", y=w343) -> (x = y?=w342:bool)
        n232 = Unbundle By Name(w325) -> ("SI camera info.Hg(Ar)"=w326:bool, "SI camera info.Cu"=w316:bool, "SI camera info.Ne"=w317:bool, "SI camera info.Bulb"=w318:bool, "SI camera info.Ar"=w319:bool, "SI camera info.Fe"=w320:bool, "SI camera info.Quartz"=w321:bool, "SI camera info.Quartz Percent"=w322:i32, "SI camera info.Dome"=w310:bool, "SI camera info.DomePercent"=w309:i32)
        n233 = case shown="True" w342 {
          tunnel: w345 -> [_ _]
          tunnel: w341 -> [_ w364]
          tunnel: [errorcluster {"status"=TRUE, "code"=0, "source"="Lamps"} ("error constant") w364] -> w353
          frame False {
          }
          frame True {
            # "Command Recieved\nwithout error yay"
            n234 = Wait (ms)(milliseconds to wait=10000) -> ()  [unwired: 1 out]
          }
        }
        n235 = local read "Current Lamp cluster"() -> (w324:T1)
        n236 = Bundle By Name(cluster=w324, "Hg(Ar)"=w326, "Cu"=w316, "Ne"=w317, "Bulb"=w318, "Ar"=w319, "Fe"=w320, "Quartz"=w321, "Current Quartz Percent"=w322, "Dome"=w310, "Dome Percent"=w309) -> (w323:T1)
        n237 = local write "Current Lamp cluster"(w323) -> ()
      }
      frame "Mirror" {
        (unwired) FALSE
        # "Wait for the comp mirror \nto be in the correct state"
        # "If we have a lamp pause\nand are using lamps then \nwe want the mirror in\nand vice versa"
        # "Wait for acknowledgement"
        # "Send to server"
        n238 = Unbundle By Name(w369) -> ("Comp mirror in?"=w368:bool)
        n239 = Select(t="IN", s=w368, f="OUT") -> (s? t:f=w371:string)
        n240 = Build Array(w371) -> (w370:string[])
        n241 = local read "Script"() -> (w366:T2)
        n242 = Bundle By Name(cluster=w366, "Lamp Pause"=FALSE) -> (w367:T2)
        n243 = call "FormCommand2.vi"("Parameters"=w370, "Command"="MIRROR") -> ("Command string"=w375:string)
        n244 = call "TCP Write with Size.vi"("error in (no error)"=w386, "data in"=w375, "connection ID"=w388) -> ("error out"=w382:errorcluster, "connection ID out"=w383:refnum<k5>)  [unwired: 6 in, 1 out]
        n245 = local write "Script"(w367) -> ()
        n246 = call "TCP Read with Size.vi"("error in (no error)"=w382, "timeout ms (25000)"=2000, "connection ID"=w383) -> ("error out"=w377:errorcluster, "data out"=w384:string)  [unwired: 6 in, 1 out]
        n247 = while {
          tunnel: w368 -> [w390]
          stop <- w389 stop-if-true
          # "add timeout break here"
          n248 = global read "TCSLINK_global.vi" "Comp Mirror"() -> (w391:bool)
          n249 = Equal?(x=w391, y=w390) -> (x = y?=w389:bool)
        }
        n250 = call "ParseCommand.vi"("Command string"=w384) -> ("Command"=w379:string, "Parameters"=w381:string[])
        n251 = Equal?(x="OK", y=w379) -> (x = y?=w378:bool)
        n252 = case shown="False" w378 {
          tunnel: w381 -> [_ _]
          tunnel: w377 -> [_ w393]
          tunnel: [errorcluster {"status"=TRUE, "code"=0, "source"="Lamps"} ("error constant") w393] -> w387
          frame False {
          }
          frame True {
            # "Command Recieved\nwithout error yay"
          }
        }
      }
      frame "Change Setup" {
        (unwired) FALSE
        # "make setup check more robust"
        # "Valid Setup?"
        # "Wait for acknowledgement"
        # "If setup needs to be changed, change setup"
        n253 = local read "Current Line"() -> (w422:dbl)
        n254 = Index Array(array=w423, index=w422) -> (element=w410:T8)
        n255 = Unbundle By Name(w410) -> ("Configuration.Name"=w417:string)
        n256 = local read "Setup Names"() -> (w416:string[])
        n257 = Search 1D Array(1D array=w416, element=w417) -> (index of element=w414:i32)  [unwired: 1 in]
        n258 = local read "Setups"() -> (w415:T5)
        n259 = Index Array(array=w415, index=w414) -> (element=w413:T9)
        n260 = local read "Script"() -> (w399:T2)
        n261 = Unbundle By Name(w413) -> ("Focus Value"=w411:dbl, "Focus Test updated?"=w412:bool)
        n262 = case shown="False" w412 {
          tunnel: w411 -> [_ w426]
          tunnel: w410 -> [w424 w427]
          tunnel: [w424 w425] -> w409
          frame False {
            # "If the value hasnt been focus test updated,\njust send whatever was entered in script"
          }
          frame True {
            # "If the focus test has been run,\nuse tested focus for this setup name"
            n263 = Bundle By Name(cluster=w427, "Configuration.Camera Focus"=w426) -> (w425:T8)
          }
        }
        n264 = Unbundle By Name(w409) -> ("Configuration"=w395:T10)
        n265 = Unbundle By Name(w395) -> ("Slit Mask"=w401:string)
        n266 = call "InstConfigToSetupStr.vi"("Configuration"=w395) -> ("Command"=w396:string)  [unwired: 10 in]
        n267 = Not Equal?(x="<NO SLIT>", y=w401) -> (x != y?=w397:bool)
        n268 = Bundle By Name(cluster=w399, "Using a slit?"=w397) -> (w398:T2)
        n269 = call "TCP Write with Size.vi"("error in (no error)"=w394, "data in"=w396, "connection ID"=w421) -> ("error out"=w404:errorcluster, "connection ID out"=w405:refnum<k5>)  [unwired: 6 in, 1 out]
        n270 = local write "Script"(w398) -> ()
        n271 = call "TCP Read with Size.vi"("error in (no error)"=w404, "timeout ms (25000)"=2000, "connection ID"=w405) -> ("error out"=w418:errorcluster, "data out"=w406:string)  [unwired: 6 in, 1 out]
        n272 = call "ParseCommand.vi"("Command string"=w406) -> ("Command"=w403:string)  [unwired: 1 out]
        n273 = Equal?(x="OK", y=w403) -> (x = y?=w419:bool)
        n274 = case shown="True" w419 {
          tunnel: w418 -> [_ w429]
          tunnel: [errorcluster {"status"=TRUE, "code"=0, "source"="Invalid Setup"} ("error constant") w429] -> w420
          frame False {
          }
          frame True {
            # "Command Recieved\nwithout error yay"
          }
        }
      }
      frame "Change SI" {
        (unwired) FALSE
        # "Wait for acknowledgement"
        # "Send to server"
        # "unpackage Si commands to string"
        n275 = local read "Current Line"() -> (w442:dbl)
        n276 = Index Array(array=w446, index=w442) -> (element=w445:T8)
        n277 = Unbundle By Name(w445) -> ("SI camera info"=w441:T11)
        n278 = call "SiConfigToCamsetStr.vi"("error in (no error)"=w433, "SI camera info"=w441) -> ("error out"=w439:errorcluster, "Command String"=w440:string)  [unwired: 8 in]
        n279 = call "TCP Write with Size.vi"("error in (no error)"=w439, "data in"=w440, "connection ID"=w443) -> ("error out"=w438:errorcluster, "connection ID out"=w444:refnum<k5>)  [unwired: 6 in, 1 out]
        n280 = call "TCP Read with Size.vi"("error in (no error)"=w438, "timeout ms (25000)"=2000, "connection ID"=w444) -> ("error out"=w432:errorcluster, "data out"=w447:string)  [unwired: 6 in, 1 out]
        n281 = call "ParseCommand.vi"("Command string"=w447) -> ("Command"=w435:string, "Parameters"=w437:string[])
        n282 = Equal?(x="OK", y=w435) -> (x = y?=w434:bool)
        n283 = case shown="True" w434 {
          tunnel: w437 -> [_ _]
          tunnel: w432 -> [_ w450]
          tunnel: [errorcluster {"status"=TRUE, "code"=0, "source"="Change SI"} ("error constant") w450] -> w431
          frame False {
          }
          frame True {
            # "Command Recieved\nwithout error yay"
          }
        }
      }
      frame "Target" {
        (unwired) FALSE
        # "Update current target with ordered target"
        # "Wait for acknowledgement"
        # "Send to server"
        n284 = local read "Current Line"() -> (w467:dbl)
        n285 = Index Array(array=w471, index=w467) -> (element=w470:T8)
        n286 = Unbundle By Name(w470) -> ("RA (HH:MM:SS.SS)"=w453:string, "DEC (HH:MM:SS.SS)"=w452:string)
        n287 = Build Array(w453, w452) -> (w456:string[])
        n288 = call "FormCommand2.vi"("Parameters"=w456, "Command"="TARGET") -> ("Command string"=w455:string)
        n289 = local read "Current Target"() -> (w454:cluster{"RA":string, "DEC":string})
        n290 = call "TCP Write with Size.vi"("error in (no error)"=w457, "data in"=w455, "connection ID"=w468) -> ("error out"=w466:errorcluster, "connection ID out"=w469:refnum<k5>)  [unwired: 6 in, 1 out]
        n291 = Bundle By Name(cluster=w454, "RA"=w453, "DEC"=w452) -> (w451:cluster{"RA":string, "DEC":string})
        n292 = local write "Current Target"(w451) -> ()
        n293 = call "TCP Read with Size.vi"("error in (no error)"=w466, "timeout ms (25000)"=2000, "connection ID"=w469) -> ("error out"=w461:errorcluster, "data out"=w472:string)  [unwired: 6 in, 1 out]
        n294 = call "ParseCommand.vi"("Command string"=w472) -> ("Command"=w463:string, "Parameters"=w465:string[])
        n295 = Equal?(x="OK", y=w463) -> (x = y?=w462:bool)
        n296 = case shown="True" w462 {
          tunnel: w465 -> [_ _]
          tunnel: w461 -> [_ w475]
          tunnel: [errorcluster {"status"=TRUE, "code"=0, "source"="Change SI"} ("error constant") w475] -> w460
          frame False {
          }
          frame True {
            # "Command Recieved\nwithout error yay"
          }
        }
      }
      frame "Focus" {
        (unwired) FALSE
        # "Wait for acknowledgement"
        # "Send to server"
        n297 = local read "Current Line"() -> (w494:dbl)
        n298 = Index Array(array=w498, index=w494) -> (element=w497:T8)
        n299 = Unbundle By Name(w497) -> ("SI camera info.Start"=w484:dbl, "SI camera info.Delta"=w479:dbl, "SI camera info.Steps"=w478:dbl)
        n300 = Number To Fractional String(number=w478) -> (F-format string=w476:string)  [unwired: 3 in]
        n301 = Number To Fractional String(number=w479) -> (F-format string=w477:string)  [unwired: 3 in]
        n302 = Number To Fractional String(number=w484) -> (F-format string=w483:string)  [unwired: 3 in]
        n303 = Build Array(w483, w477, w476) -> (w482:string[])
        n304 = call "FormCommand2.vi"("Parameters"=w482, "Command"="FOCUS") -> ("Command string"=w481:string)
        n305 = call "TCP Write with Size.vi"("error in (no error)"=w480, "data in"=w481, "connection ID"=w495) -> ("error out"=w493:errorcluster, "connection ID out"=w496:refnum<k5>)  [unwired: 6 in, 1 out]
        n306 = call "TCP Read with Size.vi"("error in (no error)"=w493, "timeout ms (25000)"=2000, "connection ID"=w496) -> ("error out"=w488:errorcluster, "data out"=w499:string)  [unwired: 6 in, 1 out]
        n307 = call "ParseCommand.vi"("Command string"=w499) -> ("Command"=w490:string, "Parameters"=w492:string[])
        n308 = Equal?(x="OK", y=w490) -> (x = y?=w489:bool)
        n309 = case shown="True" w489 {
          tunnel: w492 -> [_ _]
          tunnel: w488 -> [_ w502]
          tunnel: [errorcluster {"status"=TRUE, "code"=0, "source"="Change SI"} ("error constant") w502] -> w487
          frame False {
          }
          frame True {
            # "Command Recieved\nwithout error yay"
          }
        }
      }
      frame "SetupUpdateFocus" {
        # "update focus value \nafter focus test"
        n310 = local read "Current Setup Name"() -> (w505:string)
        n311 = local read "Setup Names"() -> (w514:string[])
        n312 = Search 1D Array(1D array=w514, element=w505) -> (index of element=w507:i32)  [unwired: 1 in]
        n313 = local read "Setups"() -> (w513:T5)
        n314 = Index Array(array=w513, index=w507) -> (element=w508:T9)
        n315 = call "Focus Test Results"() -> ("Focus Value"=w506:dbl, "OK"=w512:bool)  [unwired: 17 in, 1 out]
        n316 = Bundle By Name(cluster=w508, "Setup Name"=w505, "Focus Test updated?"=w512, "Focus Value"=w506) -> (w511:T9)
        n317 = local read "Setups"() -> (w509:T5)
        n318 = Replace Array Subset(array=w509, new element=w511, index=w507) -> (w510:T5)
        n319 = local write "Setups"(w510) -> ()
      }
      frame "Start" {
        (unwired) FALSE
        # "Wait for acknowledgement"
        # "Send to server"
        # "This is where command to start exposure happens"
        n320 = call "TCP Write with Size.vi"("error in (no error)"=w519, "data in"="START", "connection ID"=w518) -> ("error out"=w525:errorcluster, "connection ID out"=w526:refnum<k5>)  [unwired: 6 in, 1 out]
        n321 = call "TCP Read with Size.vi"("error in (no error)"=w525, "timeout ms (25000)"=2000, "connection ID"=w526) -> ("error out"=w520:errorcluster, "data out"=w527:string)  [unwired: 6 in, 1 out]
        n322 = call "ParseCommand.vi"("Command string"=w527) -> ("Command"=w522:string, "Parameters"=w524:string[])
        n323 = Equal?(x="OK", y=w522) -> (x = y?=w521:bool)
        n324 = case shown="False" w521 {
          tunnel: w524 -> [_ _]
          tunnel: w520 -> [_ w530]
          tunnel: [errorcluster {"status"=TRUE, "code"=0, "source"="Start Exposure"} ("error constant") w530] -> w516
          frame False {
          }
          frame True {
            # "Command Recieved\nwithout error yay"
          }
        }
      }
      frame "Abort" {
        (unwired) FALSE
        # "Wait for acknowledgement"
        # "Send to server"
        # "Pause = yes"
        # "Send Abort Command, Abort command should pause the Script"
        n325 = call "TCP Write with Size.vi"("error in (no error)"=w533, "data in"="ABORT", "connection ID"=w534) -> ("error out"=w542:errorcluster, "connection ID out"=w543:refnum<k5>)  [unwired: 6 in, 1 out]
        n326 = local write "Pause Button"(TRUE) -> ()
        n327 = call "TCP Read with Size.vi"("error in (no error)"=w542, "timeout ms (25000)"=2000, "connection ID"=w543) -> ("error out"=w537:errorcluster, "data out"=w544:string)  [unwired: 6 in, 1 out]
        n328 = call "ParseCommand.vi"("Command string"=w544) -> ("Command"=w539:string, "Parameters"=w541:string[])
        n329 = Equal?(x="OK", y=w539) -> (x = y?=w538:bool)
        n330 = case shown="False" w538 {
          tunnel: w541 -> [_ _]
          tunnel: w537 -> [_ w547]
          tunnel: [errorcluster {"status"=TRUE, "code"=0, "source"="Abort Exposure"} ("error constant") w547] -> w535
          frame False {
          }
          frame True {
            # "Command Recieved\nwithout error yay"
          }
        }
      }
      frame "SYSTEM_POS" {
        (unwired) FALSE
        # "Wait for acknowledgement"
        # "Send to server"
        n331 = call "TCP Write with Size.vi"("error in (no error)"=w550, "data in"="SYSTEM_POS", "connection ID"=w551) -> ("error out"=w558:errorcluster, "connection ID out"=w559:refnum<k5>)  [unwired: 6 in, 1 out]
        n332 = call "TCP Read with Size.vi"("error in (no error)"=w558, "timeout ms (25000)"=2000, "connection ID"=w559) -> ("error out"=w554:errorcluster, "data out"=w560:string)  [unwired: 6 in, 1 out]
        n333 = call "ParseCommand.vi"("Command string"=w560) -> ("Command"=w556:string, "Parameters"=w549:string[])
        n334 = for {
          tunnel: w549 -> [w562] mode=indexing
          i -> [w563]
          n335 = case shown="8" w563 {
            tunnel: w562 -> [w565 w567 w569 w571 w572 w573 w574 w575 w576]
            frame 0, Default {
              n336 = Decimal String To Number(string=w565) -> (number=→"Coll Position":i32)  [unwired: 2 in, 1 out]
            }
            frame 1 {
              n337 = Decimal String To Number(string=w567) -> (number=→"Camera Angle":i32)  [unwired: 2 in, 1 out]
            }
            frame 2 {
              n338 = Decimal String To Number(string=w569) -> (number=→"Grating Angle":i32)  [unwired: 2 in, 1 out]
            }
            frame 3 {
              n339 = Decimal String To Number(string=w571) -> (number=→"Camera Focus":i32)  [unwired: 2 in, 1 out]
            }
            frame 4 {
              "Grating" <- w572
            }
            frame 5 {
              "Slit" <- w573
            }
            frame 6 {
              "Primary Filter" <- w574
            }
            frame 7 {
              "Secondary Filter" <- w575
            }
            frame 8 {
              "Wavelength Mode" <- w576
            }
          }
        }
        n340 = Equal?(x="OK", y=w556) -> (x = y?=w555:bool)
        n341 = case shown="True" w555 {
          tunnel: w549 -> [_ _]
          tunnel: w554 -> [_ w578]
          tunnel: [errorcluster {"status"=TRUE, "code"=0, "source"="System Position"} ("error constant") w578] -> w552
          frame False {
          }
          frame True {
          }
        }
      }
      frame "TEST" {
        (unwired) FALSE
        # "Send a test command"
        # "Wait for acknowledgement"
        # "Send to server"
        n342 = call "TCPWriteWithSize.vi"("error in (no error)"=w586, "Command String"="TEST", "Connection In"=w587) -> ("error out"=w581:errorcluster, "Connection out"=w584:refnum<k5>)  [unwired: 7 in]
        n343 = call "TCPReadWithSize.vi"("error in (no error)"=w581, "Timeout ms"=2000 ("timeout ms (25000)"), "Connection In"=w584) -> ("error out"=w582:errorcluster, "Command String"=w583:string)  [unwired: 6 in, 1 out]
        n344 = call "ParseCommand.vi"("Command string"=w583) -> ("Command"=w590:string, "Parameters"=w592:string[])
        n345 = Equal?(x="OK", y=w590) -> (x = y?=w589:bool)
        n346 = case shown="True" w589 {
          tunnel: w592 -> [_ _]
          tunnel: w582 -> [_ w594]
          tunnel: [errorcluster {"status"=TRUE, "code"=0, "source"="Abort Exposure"} ("error constant") w594] -> w588
          frame False {
          }
          frame True {
            # "Command Recieved\nwithout error yay"
          }
        }
      }
      frame "Init" {
        (unwired) FALSE
        # "open GSS"
        n347 = Current VI's Path() -> (path=w604:path)
        n348 = Strip Path(path=w604) -> (stripped path=w600:path)  [unwired: 1 out]
        n349 = invoke on="Array" class="Arr (strict)" method="Reinit To Default"() -> ()  [unwired: 3 in, 3 out]
        n350 = invoke on="Total Cluster" class="Arr (strict)" method="Reinit To Default"() -> ()  [unwired: 3 in, 3 out]
        n351 = Build Path(base path=w600, name or relative path="TCPServer\\GSCS_Server.vi") -> (appended path=w601:path)
        n352 = Open VI Reference(vi path=w601) -> (vi reference=w597:refnum<vi>)  [unwired: 5 in, 1 out]
        n353 = invoke on="Script location" class="Path" method="Reinit To Default"() -> ()  [unwired: 3 in, 3 out]
        n354 = invoke on="Script" class="Clust (strict)" method="Reinit To Default"() -> ()  [unwired: 3 in, 3 out]
        n355 = invoke class="VI" method="FP.Open"(reference=w597, "State"=3) -> (reference out=w596:refnum<vi>)  [unwired: 3 in, 4 out]
        n356 = invoke on="Current Lamp cluster" class="Clust (strict)" method="Reinit To Default"() -> ()  [unwired: 3 in, 3 out]
        n357 = invoke on="Current Line" class="DigNum (strict)" method="Reinit To Default"() -> ()  [unwired: 3 in, 3 out]
        n358 = invoke class="VI" method="Run VI"(reference=w596, "Wait until done"=FALSE) -> (reference out=w602:refnum<vi>)  [unwired: 3 in, 4 out]
        n359 = Close Reference(reference=w602) -> ()  [unwired: 1 in, 1 out]
      }
      frame "Init TCP" {
        (unwired) FALSE
        (unwired) "GSS"
        # "Init tcp connection"
        n360 = TCP Open Connection(remote port or service name=u16 6969, error in (no error)=w612) -> (connection ID=w607:refnum<k5>, error out=w611:errorcluster)  [unwired: 3 in]
        n361 = local write "TCP Connection ID"(w607) -> ()
        n362 = case shown="No Error" w611 {
          selector: w611 -> [w613 _]
          tunnel: [w613 w614] -> w610
          tunnel: w609 -> [_ w615]
          frame No Error {
          }
          frame Error {
            n363 = Enqueue Element(queue=w615, element=cluster{string, string} {"Init", ""}) -> (error out=w614:errorcluster)  [unwired: 2 in, 2 out]
          }
        }
      }
      frame "ERROR" {
        (unwired) FALSE
        n364 = Unbundle(w625) -> ("source"=w624:string)  [unwired: 2 out]
        n365 = case shown="\"\", Default" w624 {
          selector: w624 -> [w631 _ _ _]
          tunnel: [w631 "An Error occured while attempting to send Camera Settings " "An Error occured while attempting to send Configuration Parameters " "An Error occured while attempting to send lamp settings "] -> w618
          frame "", Default {
          }
          frame "Change SI" {
          }
          frame "Invalid Setup" {
          }
          frame "Lamps" {
          }
        }
        n366 = Two Button Dialog(message=w618, 1:"Quit", 2:"Continue") -> (T button?=w621:bool)
        n367 = case shown="True" w621 {
          selector: w621 -> [_ w629]
          tunnel: w620 -> [w627 _]
          tunnel: [w626 errorcluster {"status"=FALSE, "code"=0, "source"=""} ("error constant")] -> w619
          frame False {
            n368 = Enqueue Element(queue=w627, element=cluster{string, string} {"QUIT", ""}) -> (error out=w626:errorcluster)  [unwired: 2 in, 2 out]
          }
          frame True {
            # "Continue"
            n369 = local write "Pause Button"(w629) -> ()
          }
        }
      }
      frame "SHUTDOWN" {
        # "Wait for acknowledgement"
        # "Send to server"
        n370 = call "TCP Write with Size.vi"("error in (no error)"=w637, "data in"="QUIT", "connection ID"=w636) -> ("error out"=w645:errorcluster, "connection ID out"=w646:refnum<k5>)  [unwired: 6 in, 1 out]
        n371 = call "TCP Read with Size.vi"("error in (no error)"=w645, "timeout ms (25000)"=2000, "connection ID"=w646) -> ("error out"=w640:errorcluster, "data out"=w647:string)  [unwired: 6 in, 1 out]
        n372 = call "ParseCommand.vi"("Command string"=w647) -> ("Command"=w642:string, "Parameters"=w644:string[])
        n373 = Equal?(x="OK", y=w642) -> (x = y?=w641:bool)
        n374 = case shown="True" w641 {
          tunnel: w644 -> [_ _]
          tunnel: w640 -> [_ w650]
          tunnel: [errorcluster {"status"=TRUE, "code"=0, "source"="QUIT"} ("error constant") w650] -> w638
          frame False {
          }
          frame True {
            # "Command Recieved\nwithout error yay"
          }
        }
      }
    }
    n375 = Equal?(x=w8, y="CLOSE") -> (x = y?=w7:bool)
  }
